vi "Path to PGSQL Configuration File.vi"(11 "Application":enum16{"TC", "FP"}(ring)) -> (3 "appended path":path)   [LabVIEW 2019, in "FP-TC-Shared.lvclass"]
uses:
  FP-TC-Shared.lvclass
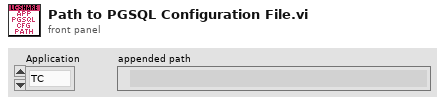
[diagram p1: front panel]
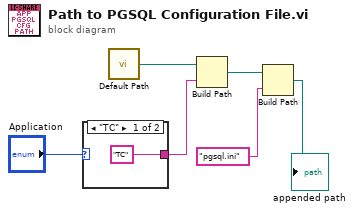
[diagram p0: block diagram]
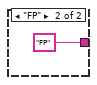
[diagram p2: hidden frame]
diagram:
  n1 = case shown="\"TC\"" "Application" {
    tunnel: ["TC" ("name or relative path") "FP" ("name or relative path")] -> w3
    frame "TC" {
    }
    frame "FP" {
    }
  }
  n2 = call "Default Path.vi"() -> ("base path"=w2:path)
  n3 = Build Path(base path=w2, name or relative path=w3) -> (appended path=w4:path)
  n4 = Build Path(base path=w4, name or relative path="pgsql.ini") -> (appended path=→"appended path":path)
